vi "jettl.vi"(0 "Path":path, 4 "Creator":refnum<user-event>, 6 "Creator Alias":string, 8 "Self Alias":string, 9 "Queue of Init":refnum<queue>, 10 "jettl":refnum<class "jettl.lvclass">) -> ()   [LabVIEW 2021, in "jettl.lvlib" / "Base jettl.lvclass"]
uses:
  Base jettl.lvclass
  jettl/jettl.lvclass
  Msg Strategy/Msg Strategy.lvclass
  C:/git/jettl/jettl/jettl/jettl/jettl.lvclass
  Base jettl.lvclass/Base jettl.ctl
  Addresses Strategy/Addresses Strategy.lvlib
  Last Ack Msg Strategy/Last Ack Msg Strategy.lvlib
  Init.ctl
  C:/git/jettl/jettl/Create Msg Strategy/Create/Create.lvclass
  C:/git/jettl/jettl/jettl/Last Ack Msg Strategy/Last Ack/Last Ack.lvclass
  C:/git/jettl/jettl/Merge Error Msg Strategy/Merge Error/Merge Error.lvclass
  C:/git/jettl/jettl/Override Error Msg Strategy/Override Error/Override Error.lvclass
  C:/git/jettl/jettl/Setup Msg Strategy/Setup/Setup.lvclass
  C:/git/jettl/jettl/Teardown Msg Strategy/Teardown/Teardown.lvclass
  C:/git/jettl/jettl/jettl/Base jettl/Base jettl.lvclass
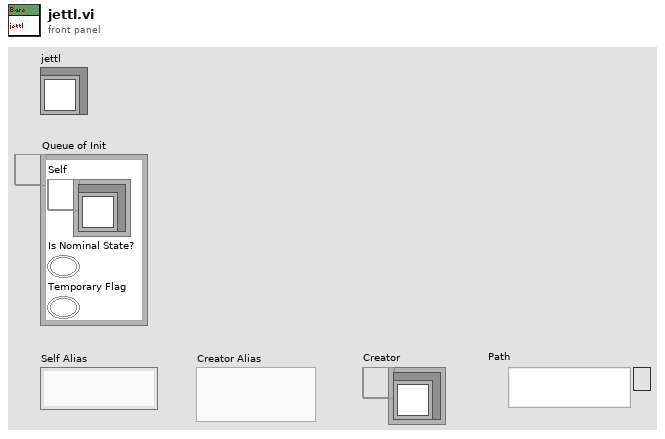
[diagram p1: front panel]
types:
  T1 = typedef "jettl.lvlib/Base jettl.lvclass/Init.ctl" = cluster{"Self":refnum<user-event>, "Is Nominal State?":bool, "Temporary Flag":bool}
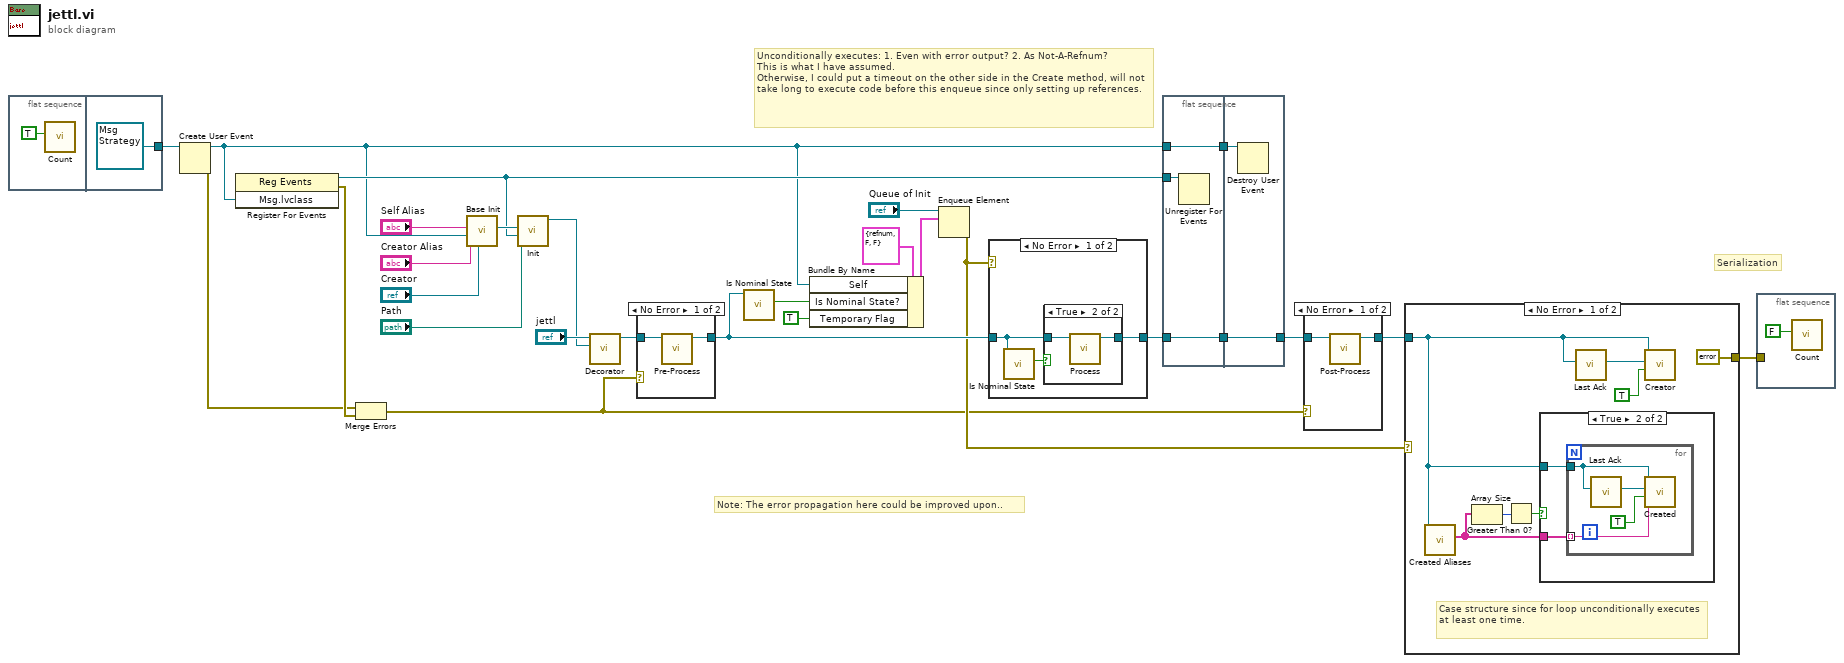
[diagram p0: block diagram]
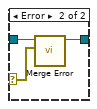
[diagram p2: hidden frame]
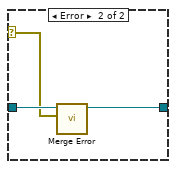
[diagram p7: hidden frame]
diagram:
  # "Note: The error propagation here could be improved upon.."
  # "Serialization"
  # "Unconditionally executes: 1. Even with error output? 2. As Not-A-Refnum?\nThis is what I have assumed.\nOtherwise, I could put a timeout on the other side in the Create method, will not take long to execute code before this enqueue since only setting up references."
  n1 = flat-sequence {
    tunnel: [refnum<class "Msg Strategy.lvclass"> refnum ("Msg.lvclass")] -> w21
    frame #0 {
      n2 = call "Count.vi"("Increment?"=TRUE) -> ()  [unwired: 11 in]
    }
    frame #1 {
    }
  }
  n3 = Create User Event(user event datatype=w21) -> (user event=w3:refnum<user-event>, error out=w23:errorcluster)  [unwired: 1 in]
  n4 = register-events(w3) -> (reference out=w13:refnum<event-registration>, error out=w25:errorcluster)  [unwired: 2 in]
  n5 = Merge Errors(w23, w25) -> (w7:errorcluster)
  n6 = call "Base Init.vi"("Creator"="Creator", "Creator Alias"="Creator Alias", "Self"=w3, "Self Alias"="Self Alias") -> ("Addresses Strategy out"=w22:refnum<class "Addresses Strategy.lvclass">)  [unwired: 7 in]
  n7 = call "Init.vi"("Path"="Path", "Register"=w13, "Addresses Strategy"=w22) -> ("Base jettl out"=w19:refnum<class "Base jettl.lvclass">)  [unwired: 8 in]
  n8 = call-dynamic "Decorator.vi"("jettl"=w19, "jettl in"="jettl") -> ("jettl out"=w18:refnum<class "jettl.lvclass">)  [unwired: 9 in]
  n9 = case shown="No Error" w7 {
    selector: w7 -> [_ w32]
    tunnel: [w31 w33] -> w17
    tunnel: w18 -> [w30 w34]
    frame No Error {
      n10 = call-dynamic "Pre-Process.vi"("jettl in"=w30) -> ("jettl out"=w31:refnum<class "jettl.lvclass">)  [unwired: 10 in]
    }
    frame Error {
      n11 = call-dynamic "Merge Error.vi"("Error"=w32, "Merge Error in"=w34) -> ("Merge Error out"=w33:refnum<class "jettl.lvclass">)  [unwired: 9 in]
    }
  }
  n12 = call-dynamic "Is Nominal State.vi"("jettl in"=w17) -> ("Is Nominal State?"=w2:bool)  [unwired: 10 in]
  n13 = Bundle By Name(cluster=T1 {"Self"=refnum, "Is Nominal State?"=FALSE, "Temporary Flag"=FALSE} ("element"), "Self"=w3, "Is Nominal State?"=w2, "Temporary Flag"=TRUE) -> (w4:T1)
  n14 = Enqueue Element(queue="Queue of Init", element=w4) -> (error out=w9:errorcluster)  [unwired: 2 in, 2 out]
  n15 = case shown="No Error" w9 {
    selector: w9 -> [_ w41]
    tunnel: [w37 w42] -> w14
    tunnel: w17 -> [w35 w43]
    frame No Error {
      n16 = call-dynamic "Is Nominal State.vi"("jettl in"=w35) -> ("Is Nominal State?"=w36:bool)  [unwired: 10 in]
      n17 = case shown="True" w36 {
        tunnel: w35 -> [w38 w40]
        tunnel: [w38 w39] -> w37
        frame False {
        }
        frame True {
          n18 = call-dynamic "Process.vi"("jettl in"=w40) -> ("jettl out"=w39:refnum<class "jettl.lvclass">)  [unwired: 10 in]
        }
      }
    }
    frame Error {
      n19 = call-dynamic "Merge Error.vi"("Error"=w41, "Merge Error in"=w43) -> ("Merge Error out"=w42:refnum<class "jettl.lvclass">)  [unwired: 9 in]
    }
  }
  n20 = flat-sequence {
    tunnel: [w46] -> w15
    tunnel: w14 -> [w46]
    tunnel: w13 -> [w45]
    tunnel: w3 -> [w44]
    tunnel: [w44] -> w12
    tunnel: [w48] -> w16
    tunnel: w15 -> [w48]
    tunnel: w12 -> [w47]
    frame #0 {
      n21 = Unregister For Events(event registration refnum=w45) -> ()  [unwired: 1 in, 1 out]
    }
    frame #1 {
      n22 = Destroy User Event(user event=w47) -> ()  [unwired: 1 in, 1 out]
    }
  }
  n23 = case shown="No Error" w7 {
    tunnel: w16 -> [w50 w51]
    tunnel: [w49 w51] -> w10
    frame No Error {
      n24 = call-dynamic "Post-Process.vi"("jettl in"=w50) -> ("jettl out"=w49:refnum<class "jettl.lvclass">)  [unwired: 10 in]
    }
    frame Error {
    }
  }
  n25 = case shown="No Error" w9 {
    tunnel: w10 -> [w53 _]
    tunnel: [errorcluster {"status"=FALSE, "code"=0, "source"=""} ("error out") _] -> w8
    frame No Error {
      # "Case structure since for loop unconditionally executes at least one time."
      n26 = call-dynamic "Created Aliases.vi"("jettl in"=w53) -> ("Created Aliases"=w57:string[])  [unwired: 10 in]
      n27 = Array Size(array=w57) -> (size(s)=w56:i32)
      n28 = Greater Than 0?(x=w56) -> (x > 0?=w55:bool)
      n29 = case shown="True" w55 {
        tunnel: w57 -> [_ w60]
        tunnel: w53 -> [_ w59]
        frame False {
        }
        frame True {
          n30 = for {
            tunnel: w59 -> [w62]
            tunnel: w60 -> [w64] mode=indexing
            n31 = call "Last Ack.vi"("jettl"=w62) -> ("Msg Strategy"=w61:refnum<class "Msg Strategy.lvclass">)  [unwired: 10 in]
            n32 = call-dynamic "Created.vi"("Created Alias"=w64, "Priority?"=TRUE, "Msg Strategy"=w61, "jettl in"=w62) -> ()  [unwired: 7 in, 1 out]
          }
        }
      }
      n33 = call "Last Ack.vi"("jettl"=w53) -> ("Msg Strategy"=w54:refnum<class "Msg Strategy.lvclass">)  [unwired: 10 in]
      n34 = call-dynamic "Creator.vi"("Priority?"=TRUE, "Msg Strategy"=w54, "jettl in"=w53) -> ()  [unwired: 8 in, 1 out]
    }
    frame Error {
    }
  }
  n35 = flat-sequence {
    tunnel: w8 -> [_]
    frame #0 {
      n36 = call "Count.vi"("Increment?"=FALSE) -> ()  [unwired: 11 in]
    }
  }
